vi "Epoxy_SaveTimer.vi"(7 "Enum":T1, 8 "error in (no error)":errorcluster, 10 "Interval":dbl, 11 "Save?":bool) -> (0 "error out":errorcluster, 1 "Int Lap [s]":dbl, 2 "Int Done?":bool, 3 "Saving?":bool)   [LabVIEW 2020]
uses:
  controls/SaveTimer.ctl
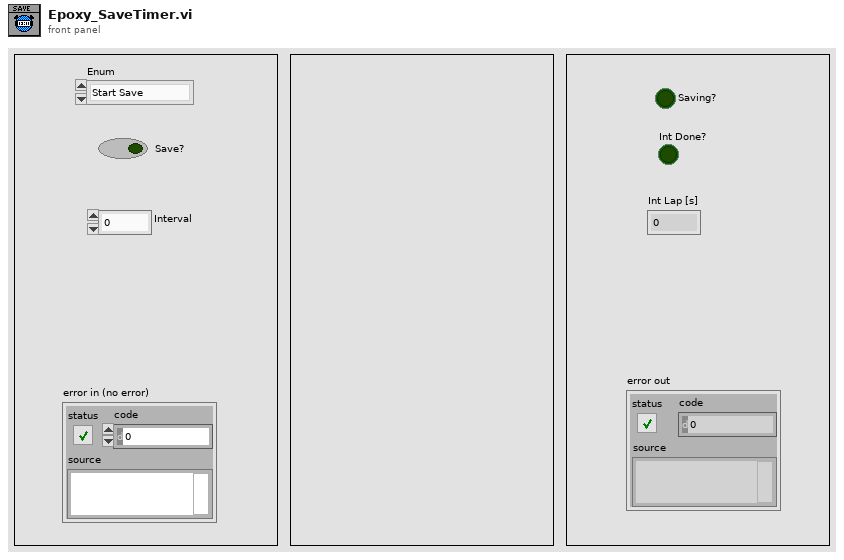
[diagram p1: front panel]
types:
  T1 = typedef "SaveTimer.ctl" = enum16{"Start Save", "StartInterval", "UpdateInterval", "Check"}
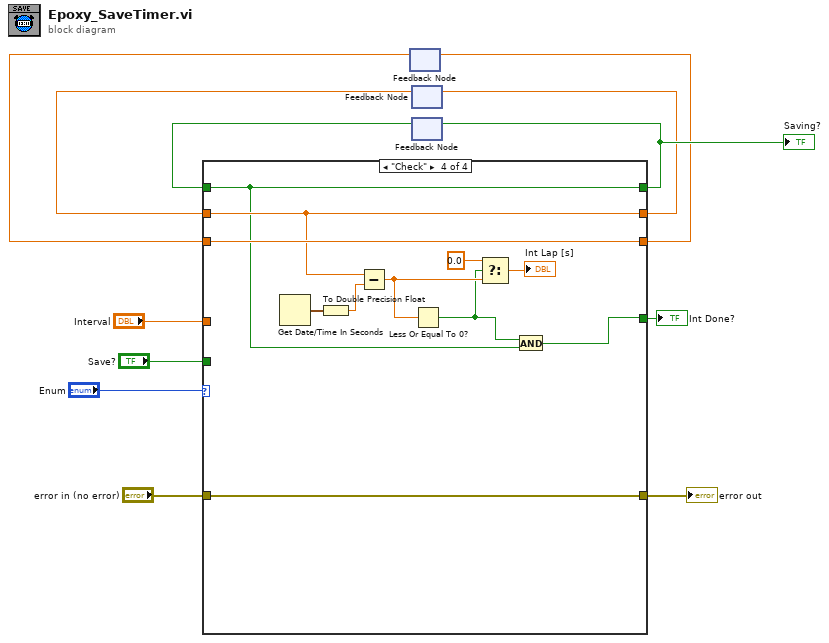
[diagram p0: block diagram]
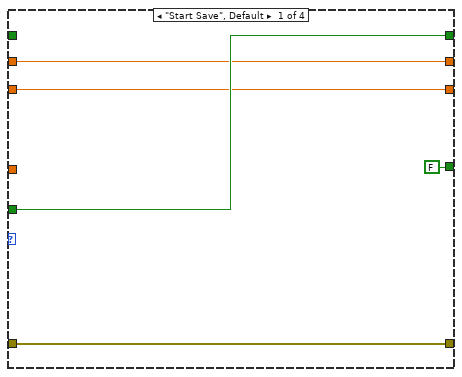
[diagram p2: hidden frame]
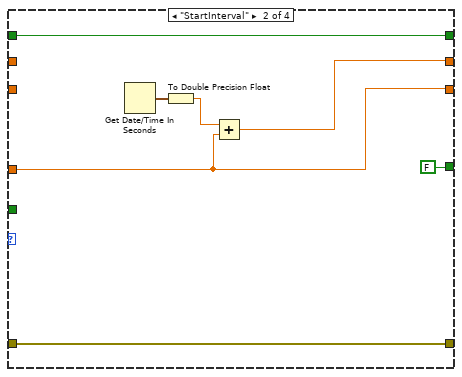
[diagram p3: hidden frame]
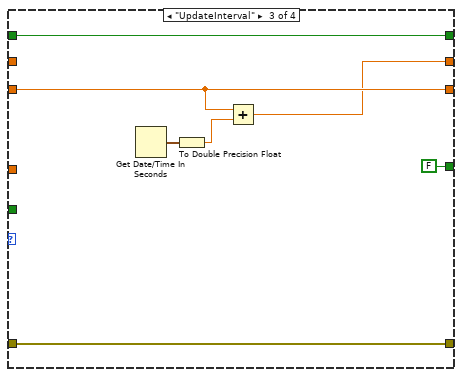
[diagram p4: hidden frame]
diagram:
  n1 = feedback #1() -> (w2:dbl)  [unwired: 1 in]
  n2 = feedback #2() -> (w4:dbl)  [unwired: 1 in]
  n3 = feedback #3() -> (w7:bool)  [unwired: 1 in]
  n4 = case shown="\"Check\"" "Enum" {
    tunnel: "error in (no error)" -> [w17 w24 w31 w42]
    tunnel: [w17 w24 w31 w42] -> w10
    tunnel: "Save?" -> [w16 _ _ _]
    tunnel: [w16 w23 w30 w34] -> w8
    tunnel: w7 -> [_ w23 w30 w34]
    tunnel: "Interval" -> [_ w19 _ _]
    tunnel: [w14 w20 w26 w39] -> w5
    tunnel: w4 -> [w14 _ _ w39]
    tunnel: [w15 w19 w28 w41] -> w3
    tunnel: w2 -> [w15 _ w28 w41]
    tunnel: [FALSE FALSE FALSE w32] -> w1
    frame "Start Save", Default {
    }
    frame "StartInterval" {
      n5 = Get Date/Time In Seconds() -> (seconds since 1Jan1904=w22:timestamp)
      n6 = To Double Precision Float(number=w22) -> (double precision float=w21:dbl)
      n7 = Add(x=w21, y=w19) -> (x+y=w20:dbl)
    }
    frame "UpdateInterval" {
      n8 = Get Date/Time In Seconds() -> (seconds since 1Jan1904=w29:timestamp)
      n9 = To Double Precision Float(number=w29) -> (double precision float=w27:dbl)
      n10 = Add(x=w28, y=w27) -> (x+y=w26:dbl)
    }
    frame "Check" {
      n11 = Get Date/Time In Seconds() -> (seconds since 1Jan1904=w40:timestamp)
      n12 = To Double Precision Float(number=w40) -> (double precision float=w38:dbl)
      n13 = Subtract(x=w39, y=w38) -> (x-y=w36:dbl)
      n14 = Less Or Equal To 0?(x=w36) -> (x <= 0?=w33:bool)
      n15 = Select(t=0.0, s=w33, f=w36) -> (s? t:f=→"Int Lap [s]":dbl)
      n16 = And(x=w33, y=w34) -> (x .and. y?=w32:bool)
    }
  }
  "error out" <- w10
  "Saving?" <- w8
  "Int Done?" <- w1
  n17 = feedback-in #1(w3) -> ()
  n18 = feedback-in #2(w5) -> ()
  n19 = feedback-in #3(w8) -> ()
